vi "_Construct.vi"(8 "error in (no error)":errorcluster, 11 "Init Parameters":T1) -> (0 "error out":errorcluster, 3 "ClashRoyale out":refnum<class "StashRoyale.lvclass">)   [LabVIEW 2020, in "StashRoyale.lvclass"]
uses:
  StashRoyale.lvclass
  <vilib>/drjdpowell/SQLite Library/SQL Connection/Connection.lvclass
  <vilib>/drjdpowell/SQLite Library/SQL Connection/Open (path).vi
  <vilib>/drjdpowell/SQLite Library/SQLite.lvlib
  <vilib>/drjdpowell/SQLite Library/SQL Connection/Execute SQL (No results).vi
  InitParameters.ctl
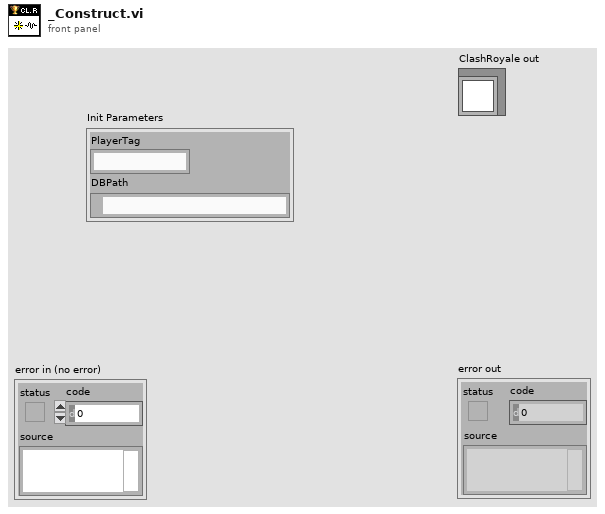
[diagram p1: front panel]
types:
  T1 = typedef "InitParameters.ctl" = cluster{"PlayerTag":string, "DBPath":path}
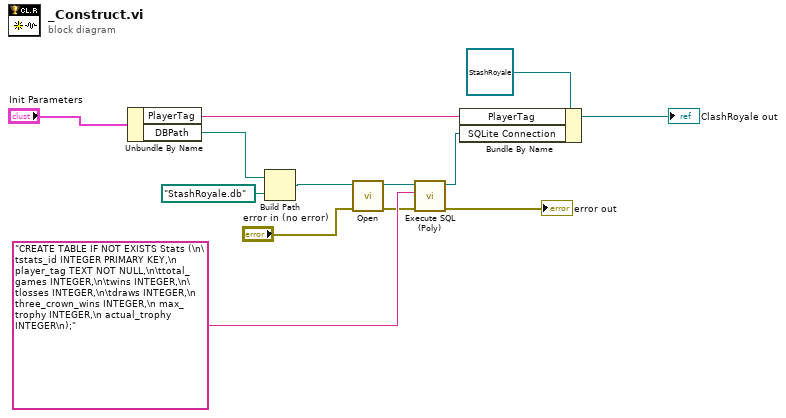
[diagram p0: block diagram]
diagram:
  n1 = Unbundle By Name("Init Parameters") -> ("PlayerTag"=w2:string, "DBPath"=w1:path)
  n2 = Build Path(base path=w1, name or relative path=path "StashRoyale.db") -> (appended path=w10:path)
  n3 = call-poly <vilib>:"Open.vi"("error in (no error)"="error in (no error)", "db file"=w10) -> ("error out"=w7:errorcluster, "SQLite Connection"=w9:refnum<class "Connection.lvclass">)  [unwired: 8 in]
  n4 = call-poly <vilib>:"Execute SQL (Poly).vi"("error in (no error)"=w7, "SQL"="CREATE TABLE IF NOT EXISTS Stats (\n\tstats_id INTEGER PRIMARY KEY,\n player_tag TEXT NOT NULL,\n\ttotal_games INTEGER,\n\twins INTEGER,\n\tlosses INTEGER,\n\tdraws INTEGER,\n three_crown_wins INTEGER,\n max_trophy INTEGER,\n actual_trophy INTEGER\n);", "SQLite Connection in"=w9) -> ("error out"=→"error out":errorcluster, "SQLite Connection"=w6:refnum<class "Connection.lvclass">)  [unwired: 7 in]
  n5 = Bundle By Name(cluster=refnum<class "StashRoyale.lvclass"> refnum ("ClashRoyale in"), "PlayerTag"=w2, "SQLite Connection"=w6) -> (→"ClashRoyale out":refnum<class "StashRoyale.lvclass">)
